vi "Begin.vi"(8 "error in":errorcluster) -> (0 "error out":errorcluster)   [LabVIEW 2018]
doc: "Called before other user functions, this VI is expected to open initial I/O refnums, load in file data, and do all program initialization. Notice that the <B>error out</B> terminal is simply used for data flow. Wiring it to other structures or subVIs ensures that this VI runs first."
uses:
  <userlib>/836-Library/System/TDMS_V2/Support/Logging_Settings.ctl
  <vilib>/Rock Robotics/WPI/DriverStation/WPI_DriverStationRobotMode2.ctl
  <vilib>/Rock Robotics/WPI/ThirdParty/Phoenix-LabVIEW/Motor Controller/Controls/CTRE_Phoenix_MotorControl_NeutralMode.ctl
  <vilib>/Rock Robotics/WPI/Solenoid/WPI_SolenoidChannel.ctl
  <vilib>/Rock Robotics/WPI/Joystick/WPI_JoystickDeviceEnum.ctl
  Robot Global Data.vi
  <vilib>/Rock Robotics/WPI/ThirdParty/Phoenix-LabVIEW/Pigeon IMU/CTRE_PigeonIMU_Open_TalonSRX.vi
  <vilib>/Rock Robotics/WPI/Solenoid/WPI_SolenoidOpenSingle.vi
  <vilib>/Rock Robotics/WPI/Utilities/WPI_GetSetVariantRefNum.vi
  <userlib>/836-Library/System/TDMS_V2/Support/Channel_Config.ctl
  <userlib>/836-Library/System/TDMS_V2/Support/Group_Config.ctl
panel:
  in  "Logging Settings":T1={"Data Grab Period"=35.0, "File Write Period"=1000.0, "Max Stored Size"=100.0, "Burst Size"=150.0}
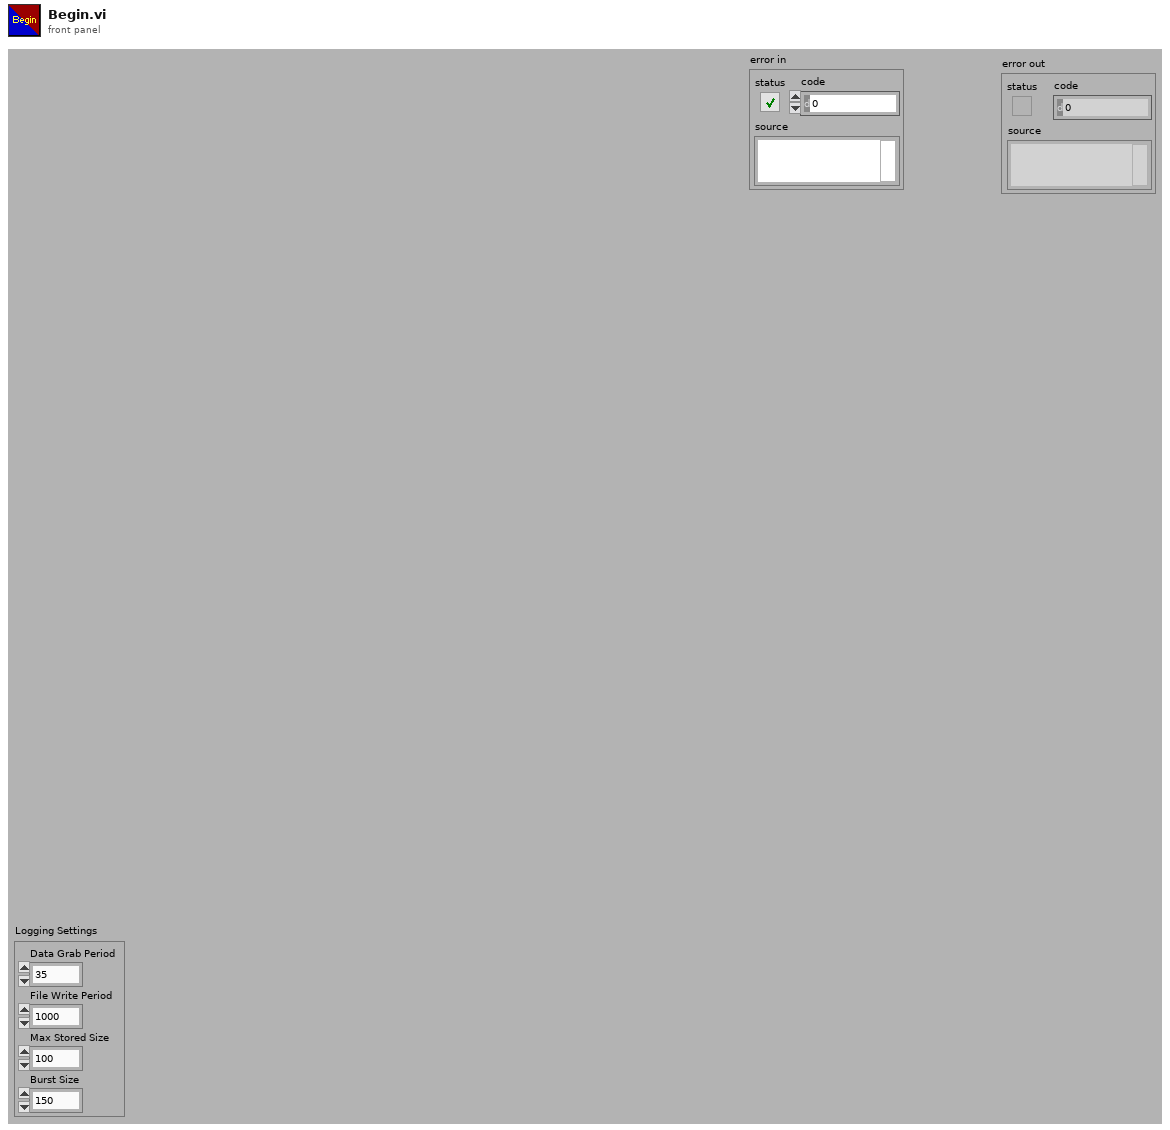
[diagram p1: front panel]
types:
  T1 = typedef "Logging_Settings.ctl" = cluster{"Data Grab Period":dbl, "File Write Period":dbl, "Max Stored Size":dbl, "Burst Size":dbl}
  T2 = typedef "WPI_SolenoidChannel.ctl" = enum8{"Solenoid 0", "Solenoid 1", "Solenoid 2", "Solenoid 3", "Solenoid 4", "Solenoid 5", "Solenoid 6", "Solenoid 7", "Invalid"}
  T3 = typedef "WPI_JoystickDeviceEnum.ctl" = enum16{"USB 0", "USB 1", "USB 2", "USB 3", "USB 4", "USB 5"}
  T4 = typedef "CTRE_Phoenix_MotorControl_NeutralMode.ctl" = enum8{"EEPROMSetting", "Override to Coast", "Override to Brake"}
  T5 = typedef "WPI_DriverStationRobotMode2.ctl" = enum16{"Autonomous Disabled", "Autonomous Enabled", "Teleop Disabled", "Teleop Enabled", "Disconnected", "Finish", "Test Disabled", "Test Enabled", "Emergency Stopped"}
  T6 = enum16{"open", "replace", "create", "open or create", "replace or create", "replace or create with confirmation"}
  T7 = typedef "Group_Config.ctl" = cluster{"Name":string, "Channel Config":T8}
  T8 = typedef "Channel_Config.ctl" = cluster{"Channel Names":string[]}
  T9 = typedef "WPI_JoystickDevRef.ctl" = cluster{"Device":T3}
  T10 = typedef "WPI_MotorControlDeviceRef.ctl" = cluster{"DeviceStatus":errorcluster, "Type":T11, "PWM":cluster{"PWM Channel":T12, "DeadBand":T13}, "CAN":cluster{"Device Number":u8, "SetOutput VI Ref":variant, "GetOutput VI Ref":variant, "Enable VI Ref":variant, "Disable VI Ref":variant, "Data":variant}, "Invert":bool, "DIO PWM":cluster{"PWM \"Enable\" Channel":T12, "DIOChannel":T14, "PWM Rate":dbl}}
  T11 = typedef "WPI_MotorControlType.ctl" = enum16{"PWM", "CAN", "DIO PWM"}
  T12 = typedef "FPGA_DIOPWMChannel.ctl" = enum8{"PWM 0", "PWM 1", "PWM 2", "PWM 3", "PWM 4", "PWM 5", "PWM 6", "PWM 7", "PWM 8", "PWM 9", "PWM MXP 0", "PWM MXP 1", "PWM MXP 2", "PWM MXP 3", "PWM MXP 4", "PWM MXP 5", "PWM MXP 6", "PWM MXP 7", "PWM MXP 8", "PWM MXP 9", "Invalid"}
  T13 = typedef "WPI_PWMDeadband.ctl" = cluster{"Name":string, "maxPositivePwm":i32, "minPositivePwm":i32, "centerPwm":i32, "maxNegativePwm":i32, "minNegativePwm":i32, "angularRange":u16}
  T14 = typedef "FPGA_DIOChannel.ctl" = enum8{"DIO 0", "DIO 1", "DIO 2", "DIO 3", "DIO 4", "DIO 5", "DIO 6", "DIO 7", "DIO 8", "DIO 9", "DIO MXP 0", "DIO MXP 1", "DIO MXP 2", "DIO MXP 3", "DIO MXP 4", "DIO MXP 5", "DIO MXP 6", "DIO MXP 7", "DIO MXP 8", "DIO MXP 9", "DIO MXP 10", "DIO MXP 11", "DIO MXP 12", "DIO MXP 13", "DIO MXP 14", "DIO MXP 15", "SPI Port CS1", "SPI Port CS2", "SPI Port CS3", "SPI Port MISO", "SPI Port MOSI", "Invalid"}
  T15 = typedef "CTRE_PigeonIMU_DeviceRef.ctl" = cluster{"DeviceStatus":errorcluster, "Device Number":u8, "Type":T16, "Device ID":u32, "Handle":u64, "UsageFrame":u32, "Library Path":path}
  T16 = typedef "CTRE_PigeonIMU_ConnectionType.ctl" = u32
  T17 = typedef "WPI_CompressorDevRef.ctl" = cluster{"DevStatus":errorcluster, "Pneumatics Control Module":u8}
  T18 = typedef "WPI_SolenoidDevRef.ctl" = cluster{"DevStatus":errorcluster, "Pneumatics Control Module":u8, "Forward Solenoid Channel":T2, "Reverse Solenoid Channel":T2}
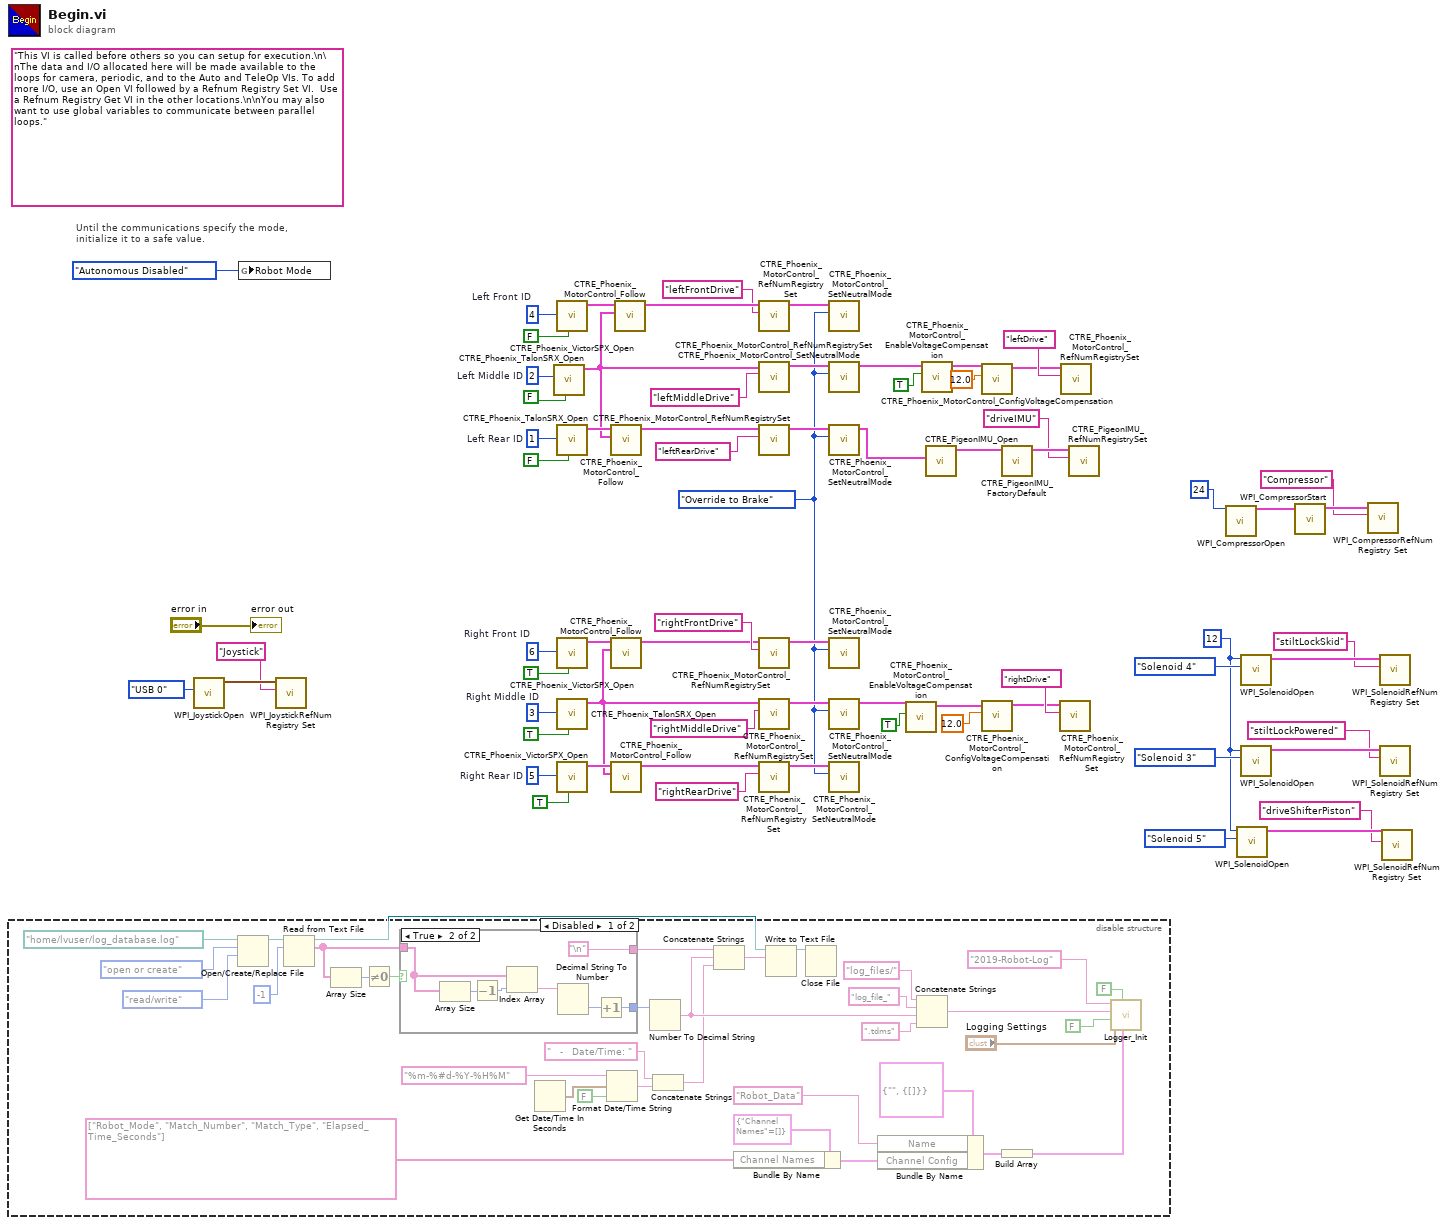
[diagram p0: block diagram]
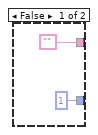
[diagram p2: hidden frame]
diagram:
  w17 = u8 12 ("Pneumatics Control Module (0)")
  w35 = CTRE_Phoenix_MotorControl_NeutralMode."Override to Brake" ("Motor Control Neutral Mode")
  w61 = u8 1  # Left Rear ID
  w51 = u8 2  # Left Middle ID
  w63 = u8 4  # Left Front ID
  w64 = u8 5  # Right Rear ID
  w66 = u8 3  # Right Middle ID
  w68 = u8 6  # Right Front ID
  (unwired) "This VI is called before others so you can setup for execution.\n\nThe data and I/O allocated here will be made available to the loops for camera, periodic, and to the Auto and TeleOp VIs. To add more I/O, use an Open VI followed by a Refnum Registry Set VI.  Use a Refnum Registry Get VI in the other locations.\n\nYou may also want to use global variables to communicate between parallel loops."
  # "Until the communications specify the mode,\ninitialize it to a safe value."
  n1 = disable-structure shown="Disabled" {
    frame Disabled {
      n2 = Open/Create/Replace File(file path (use dialog)=path "/home/lvuser/log_database.log", operation (0:open)=T6."open or create", access (0:read/write)=enum16{"read/write", "read-only", "write-only"}."read/write") -> (refnum out=w85:refnum<file>)  [unwired: 3 in, 2 out]
      n3 = Read from Text File(file (use dialog)=w85, count=-1) -> (refnum out=w78:refnum<file>, text=w84:string[])  [unwired: 2 in, 2 out]
      n4 = Array Size(array=w84) -> (size(s)=w82:i32)
      n5 = Not Equal To 0?(x=w82) -> (x != 0?=w83:bool)
      n6 = case shown="True" w83 {
        tunnel: [1 w113] -> w81
        tunnel: w84 -> [_ w112]
        tunnel: ["" "\n"] -> w80
        frame False {
        }
        frame True {
          n7 = Array Size(array=w112) -> (size(s)=w111:i32)
          n8 = Decrement(x=w111) -> (x-1=w110:i32)
          n9 = Index Array(array=w112, index=w110) -> (element=w109:string)
          n10 = Decimal String To Number(string=w109) -> (number=w114:i32)  [unwired: 2 in, 1 out]
          n11 = Increment(x=w114) -> (x+1=w113:i32)
        }
      }
      n12 = Get Date/Time In Seconds() -> (seconds since 1Jan1904=w74:timestamp)
      n13 = Format Date/Time String(time format string (%c)="%m-%#d-%Y-%H%M", seconds (now)=w74, UTC format=FALSE) -> (date/time string=w72:string)
      n14 = Number To Decimal String(number=w81) -> (decimal integer string=w77:string)  [unwired: 1 in]
      n15 = Concatenate Strings("   -   Date/Time: " ("string"), w72) -> (w73:string)
      n16 = Concatenate Strings(w80, w77, w73) -> (w79:string)
      n17 = Bundle By Name(cluster=T8 {"Channel Names"=[]} ("Channel Config"), "Channel Names"=string[] ["Robot_Mode", "Match_Number", "Match_Type", "Elapsed_Time_Seconds"]) -> (w96:T8)
      n18 = Write to Text File(file (use dialog)=w78, text=w79) -> (refnum out=w86:refnum<file>)  [unwired: 2 in, 2 out]
      n19 = Close File(refnum=w86) -> ()  [unwired: 1 in, 2 out]
      n20 = Bundle By Name(cluster=T7 {"Name"="", "Channel Config"={"Channel Names"=[]}} ("Group Config"), "Name"="Robot_Data", "Channel Config"=w96) -> (w93:T7)
      n21 = Concatenate Strings("log_files/" ("string"), "log_file_" ("TDMS Name"), w77, ".tdms" ("string")) -> (w100:string)
      n22 = Build Array(w93) -> (w92:T7[])
      n23 = call <userlib>:"Logger_Init.vi"("Group Config"=w92, "Log To Computer?"=FALSE, "Logging Settings"="Logging Settings", "Log To USB?"=FALSE, "File Name"=w100, "Logger Name"="2019-Robot-Log") -> ()  [unwired: 4 in, 2 out]
    }
    frame Enabled {
    }
  }
  n24 = call <vilib>:"WPI_JoystickOpen.vi"("JoystickDevice"=WPI_JoystickDeviceEnum."USB 0") -> ("JoystickDevRef"=w23:T9)  [unwired: 10 in]
  n25 = global write "Robot Global Data.vi" "Robot Mode"(WPI_DriverStationRobotMode2."Autonomous Disabled" ("Robot Mode")) -> ()
  n26 = call <vilib>:"WPI_JoystickRefNum Registry Set.vi"("refnum name"="Joystick", "JoystickDevRef"=w23) -> ()  [unwired: 8 in, 2 out]
  n27 = call <vilib>:"CTRE_Phoenix_TalonSRX_Open.vi"("Invert"=FALSE, "Device Number"=w51) -> ("CAN Talon SRX Ref"=w45:T10)  [unwired: 8 in, 1 out]
  n28 = call <vilib>:"CTRE_Phoenix_VictorSPX_Open.vi"("Invert"=FALSE, "Device Number"=w63) -> ("CAN Talon SRX Ref"=w48:T10)  [unwired: 8 in, 1 out]
  n29 = call <vilib>:"CTRE_Phoenix_TalonSRX_Open.vi"("Invert"=FALSE, "Device Number"=w61) -> ("CAN Talon SRX Ref"=w58:T10)  [unwired: 8 in, 1 out]
  n30 = call <vilib>:"CTRE_Phoenix_VictorSPX_Open.vi"("Invert"=TRUE, "Device Number"=w68) -> ("CAN Talon SRX Ref"=w47:T10)  [unwired: 8 in, 1 out]
  n31 = call <vilib>:"CTRE_Phoenix_TalonSRX_Open.vi"("Invert"=TRUE, "Device Number"=w66) -> ("CAN Talon SRX Ref"=w44:T10)  [unwired: 8 in, 1 out]
  n32 = call <vilib>:"CTRE_Phoenix_VictorSPX_Open.vi"("Invert"=TRUE, "Device Number"=w64) -> ("CAN Talon SRX Ref"=w59:T10)  [unwired: 8 in, 1 out]
  n33 = call <vilib>:"CTRE_Phoenix_MotorControl_Follow.vi"("Master Controller to Follow"=w45, "PhoenixMotorControlDevRef"=w58) -> ("PhoenixMotorControlDevRef"=w57:T10)  [unwired: 8 in, 1 out]
  n34 = call <vilib>:"CTRE_Phoenix_MotorControl_Follow.vi"("Master Controller to Follow"=w44, "PhoenixMotorControlDevRef"=w47) -> ("PhoenixMotorControlDevRef"=w46:T10)  [unwired: 8 in, 1 out]
  n35 = call <vilib>:"CTRE_Phoenix_MotorControl_Follow.vi"("Master Controller to Follow"=w44, "PhoenixMotorControlDevRef"=w59) -> ("PhoenixMotorControlDevRef"=w56:T10)  [unwired: 8 in, 1 out]
  n36 = call <vilib>:"CTRE_Phoenix_MotorControl_Follow.vi"("Master Controller to Follow"=w45, "PhoenixMotorControlDevRef"=w48) -> ("PhoenixMotorControlDevRef"=w49:T10)  [unwired: 8 in, 1 out]
  n37 = call <vilib>:"CTRE_Phoenix_MotorControl_RefNumRegistrySet.vi"("refnum name"="leftFrontDrive", "PhoenixMotorControlDevRef"=w49) -> ("PhoenixMotorControlDevRef"=w41:T10)  [unwired: 8 in, 1 out]
  n38 = call <vilib>:"CTRE_Phoenix_MotorControl_RefNumRegistrySet.vi"("refnum name"="leftMiddleDrive", "PhoenixMotorControlDevRef"=w45) -> ("PhoenixMotorControlDevRef"=w40:T10)  [unwired: 8 in, 1 out]
  n39 = call <vilib>:"CTRE_Phoenix_MotorControl_RefNumRegistrySet.vi"("refnum name"="leftRearDrive", "PhoenixMotorControlDevRef"=w57) -> ("PhoenixMotorControlDevRef"=w39:T10)  [unwired: 8 in, 1 out]
  n40 = call <vilib>:"CTRE_Phoenix_MotorControl_RefNumRegistrySet.vi"("refnum name"="rightFrontDrive", "PhoenixMotorControlDevRef"=w46) -> ("PhoenixMotorControlDevRef"=w38:T10)  [unwired: 8 in, 1 out]
  n41 = call <vilib>:"CTRE_Phoenix_MotorControl_RefNumRegistrySet.vi"("refnum name"="rightMiddleDrive", "PhoenixMotorControlDevRef"=w44) -> ("PhoenixMotorControlDevRef"=w37:T10)  [unwired: 8 in, 1 out]
  n42 = call <vilib>:"CTRE_Phoenix_MotorControl_RefNumRegistrySet.vi"("refnum name"="rightRearDrive", "PhoenixMotorControlDevRef"=w56) -> ("PhoenixMotorControlDevRef"=w36:T10)  [unwired: 8 in, 1 out]
  n43 = call <vilib>:"CTRE_Phoenix_MotorControl_SetNeutralMode.vi"("Motor Control Neutral Mode"=w35, "PhoenixMotorControlDevRef"=w41) -> ()  [unwired: 8 in, 2 out]
  n44 = call <vilib>:"CTRE_Phoenix_MotorControl_SetNeutralMode.vi"("Motor Control Neutral Mode"=w35, "PhoenixMotorControlDevRef"=w40) -> ("PhoenixMotorControlDevRef"=w11:T10)  [unwired: 8 in, 1 out]
  n45 = call <vilib>:"CTRE_Phoenix_MotorControl_SetNeutralMode.vi"("Motor Control Neutral Mode"=w35, "PhoenixMotorControlDevRef"=w39) -> ("PhoenixMotorControlDevRef"=w1:T10)  [unwired: 8 in, 1 out]
  n46 = call <vilib>:"CTRE_Phoenix_MotorControl_SetNeutralMode.vi"("Motor Control Neutral Mode"=w35, "PhoenixMotorControlDevRef"=w38) -> ()  [unwired: 8 in, 2 out]
  n47 = call <vilib>:"CTRE_Phoenix_MotorControl_SetNeutralMode.vi"("Motor Control Neutral Mode"=w35, "PhoenixMotorControlDevRef"=w37) -> ("PhoenixMotorControlDevRef"=w14:T10)  [unwired: 8 in, 1 out]
  n48 = call <vilib>:"CTRE_Phoenix_MotorControl_SetNeutralMode.vi"("Motor Control Neutral Mode"=w35, "PhoenixMotorControlDevRef"=w36) -> ()  [unwired: 8 in, 2 out]
  n49 = call <vilib>:"CTRE_Phoenix_MotorControl_EnableVoltageCompensation.vi"("Enable Voltage Compensation?"=TRUE, "PhoenixMotorControlDevRef"=w14) -> ("PhoenixMotorControlDevRef"=w13:T10)  [unwired: 8 in, 1 out]
  n50 = call <vilib>:"CTRE_Phoenix_MotorControl_EnableVoltageCompensation.vi"("Enable Voltage Compensation?"=TRUE, "PhoenixMotorControlDevRef"=w11) -> ("PhoenixMotorControlDevRef"=w10:T10)  [unwired: 8 in, 1 out]
  n51 = call-poly <vilib>:"CTRE_PigeonIMU_Open.vi"("CAN Talon SRX Ref"=w1) -> ("PigeonIMUDevRef"=w5:T15)  [unwired: 9 in, 1 out]
  n52 = call <vilib>:"CTRE_Phoenix_MotorControl_ConfigVoltageCompensation.vi"("Saturation Voltage"=12.0, "PhoenixMotorControlDevRef"=w10) -> ("PhoenixMotorControlDevRef"=w2:T10)  [unwired: 8 in, 1 out]
  n53 = call <vilib>:"CTRE_Phoenix_MotorControl_ConfigVoltageCompensation.vi"("Saturation Voltage"=12.0, "PhoenixMotorControlDevRef"=w13) -> ("PhoenixMotorControlDevRef"=w12:T10)  [unwired: 8 in, 1 out]
  n54 = call <vilib>:"CTRE_PigeonIMU_FactoryDefault.vi"("PigeonIMUDevRef"=w5) -> ("PigeonIMUDevRef"=w4:T15)  [unwired: 9 in, 1 out]
  n55 = call <vilib>:"CTRE_Phoenix_MotorControl_RefNumRegistrySet.vi"("refnum name"="rightDrive", "PhoenixMotorControlDevRef"=w12) -> ()  [unwired: 8 in, 2 out]
  n56 = call <vilib>:"CTRE_Phoenix_MotorControl_RefNumRegistrySet.vi"("refnum name"="leftDrive", "PhoenixMotorControlDevRef"=w2) -> ()  [unwired: 8 in, 2 out]
  n57 = call <vilib>:"CTRE_PigeonIMU_RefNumRegistrySet.vi"("refnum name"="driveIMU", "PigeonIMUDevRef"=w4) -> ()  [unwired: 8 in, 2 out]
  n58 = call <vilib>:"WPI_CompressorOpen.vi"("Pneumatics Control Module (0)"=u8 24) -> ("CompressorDevRef"=w27:T17)  [unwired: 13 in, 1 out]
  n59 = call-poly <vilib>:"WPI_SolenoidOpen.vi"("Solenoid Channel"=WPI_SolenoidChannel."Solenoid 5", "Pneumatics Control Module (0)"=w17) -> ("SolenoidDevRef"=w18:T18)  [unwired: 8 in, 1 out]
  n60 = call-poly <vilib>:"WPI_SolenoidOpen.vi"("Solenoid Channel"=WPI_SolenoidChannel."Solenoid 4", "Pneumatics Control Module (0)"=w17) -> ("SolenoidDevRef"=w33:T18)  [unwired: 8 in, 1 out]
  n61 = call-poly <vilib>:"WPI_SolenoidOpen.vi"("Solenoid Channel"=WPI_SolenoidChannel."Solenoid 3", "Pneumatics Control Module (0)"=w17) -> ("SolenoidDevRef"=w31:T18)  [unwired: 8 in, 1 out]
  n62 = call <vilib>:"WPI_CompressorStart.vi"("CompressorDevRef"=w27) -> ("CompressorDevRef"=w26:T17)  [unwired: 9 in, 1 out]
  n63 = call <vilib>:"WPI_CompressorRefNum Registry Set.vi"("refnum name"="Compressor", "CompressorDevRef"=w26) -> ()  [unwired: 8 in, 2 out]
  n64 = call <vilib>:"WPI_SolenoidRefNum Registry Set.vi"("refnum name"="stiltLockSkid", "SolenoidDevRef"=w33) -> ()  [unwired: 8 in, 2 out]
  n65 = call <vilib>:"WPI_SolenoidRefNum Registry Set.vi"("refnum name"="stiltLockPowered", "SolenoidDevRef"=w31) -> ()  [unwired: 8 in, 2 out]
  n66 = call <vilib>:"WPI_SolenoidRefNum Registry Set.vi"("refnum name"="driveShifterPiston", "SolenoidDevRef"=w18) -> ()  [unwired: 8 in, 2 out]
  "error out" <- "error in"
